vi "process_limits.vi"(10 "old output cluster":T1, 11 "Input cluster":T2) -> (0 "Update FPGA":bool, 3 "output cluster":T1)   [LabVIEW 2013]
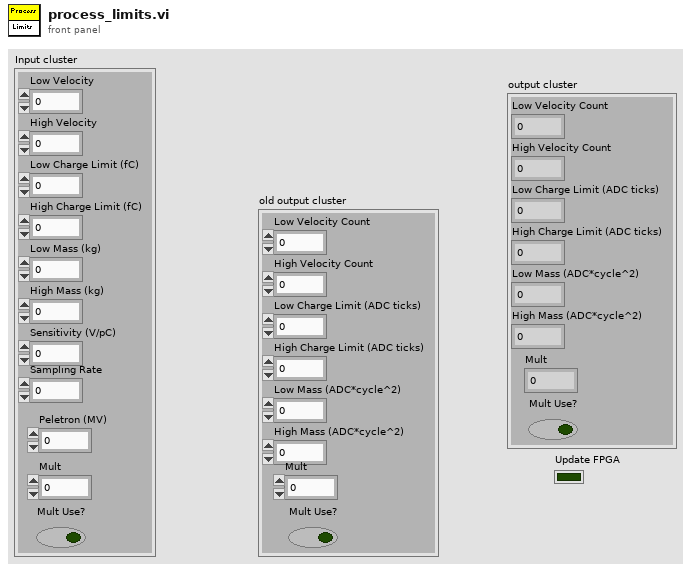
[diagram p1: front panel]
types:
  T1 = cluster{"Low Velocity Count":i32, "High Velocity Count":i32, "Low Charge Limit (ADC ticks)":i16, "High Charge Limit (ADC ticks)":i16, "Low Mass (ADC*cycle^2)":i64, "High Mass (ADC*cycle^2)":i64, "Mult":fxp<+,16,3>, "Mult Use?":bool}
  T2 = cluster{"Low Velocity":dbl, "High Velocity":dbl, "Low Charge Limit (fC)":dbl, "High Charge Limit (fC)":dbl, "Low Mass (kg)":dbl, "High Mass (kg)":dbl, "Sensitivity (V/pC)":dbl, "Sampling Rate":dbl, "Peletron (MV)":dbl, "Mult":fxp<+,16,3>, "Mult Use?":bool}
  T3 = cluster{"Low Velocity Count":i32, "High Velocity Count":i32, "Low Charge Limit (ADC ticks)":i16, "High Charge Limit (ADC ticks)":i16, "Low Mass (ADC*cycle^2)":i64, "High Mass (ADC*cycle^2)":i64}
  T4 = cluster{i32, i32, i16, i16, i64, i64, "Mult":fxp<+,16,3>, "Mult Use?":bool}
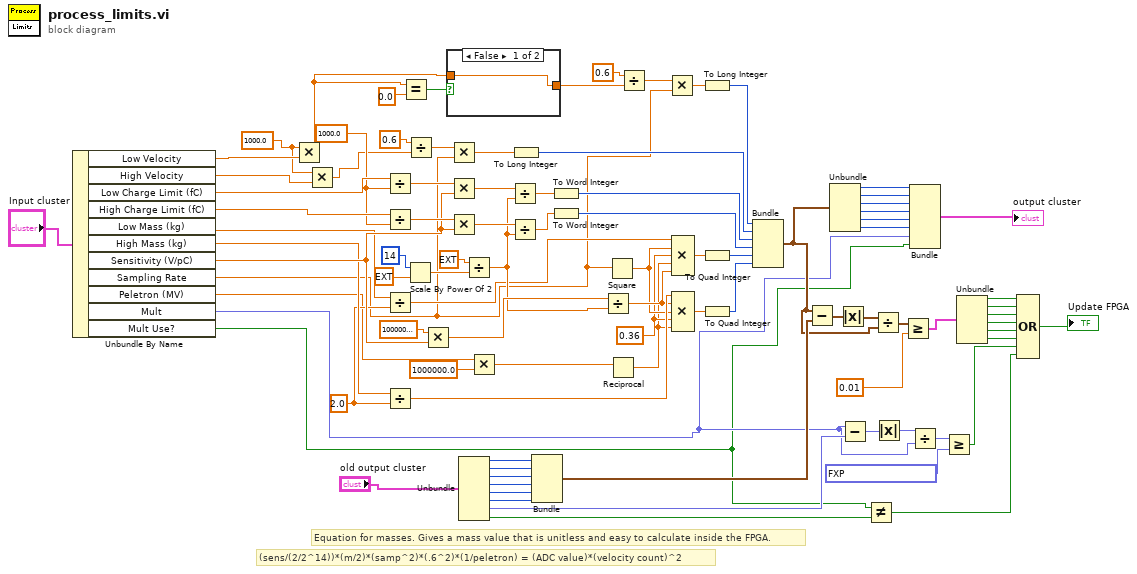
[diagram p0: block diagram]
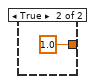
[diagram p2: hidden frame]
diagram:
  w41 = 1000.0 ("x")
  w50 = 0.36 ("value")
  w58 = 2.0 ("y")
  w71 = 1000.0 ("y")
  # "Equation for masses. Gives a mass value that is unitless and easy to calculate inside the FPGA."
  # "(sens/(2/2^14))*(m/2)*(samp^2)*(.6^2)*(1/peletron) = (ADC value)*(velocity count)^2"
  n1 = Unbundle By Name("Input cluster") -> ("Low Velocity"=w44:dbl, "High Velocity"=w42:dbl, "Low Charge Limit (fC)"=w79:dbl, "High Charge Limit (fC)"=w72:dbl, "Low Mass (kg)"=w60:dbl, "High Mass (kg)"=w59:dbl, "Sensitivity (V/pC)"=w64:dbl, "Sampling Rate"=w56:dbl, "Peletron (MV)"=w33:dbl, "Mult"=w8:fxp<+,16,3>, "Mult Use?"=w4:bool)
  n2 = Multiply(x=w41, y=w44) -> (x*y=w43:dbl)
  n3 = Multiply(x=w41, y=w42) -> (x*y=w40:dbl)
  n4 = Divide(x=w79, y=w71) -> (x/y=w78:dbl)
  n5 = Divide(x=w72, y=w71) -> (x/y=w70:dbl)
  n6 = Divide(x=w60, y=w58) -> (x/y=w57:dbl)
  n7 = Divide(x=w59, y=w58) -> (x/y=w53:dbl)
  n8 = Equal?(x=w43, y=0.0) -> (x = y?=w88:bool)
  n9 = Scale By Power Of 2(n=i16 14, x=ext 1.0) -> (x*2^n=w75:ext)
  n10 = Divide(x=0.6, y=w40) -> (x/y=w82:dbl)
  n11 = Multiply(x=1000000000000.0, y=w64) -> (x*y=w62:dbl)
  n12 = case shown="False" w88 {
    tunnel: [w92 1.0 ("y")] -> w87
    tunnel: w43 -> [w92 _]
    frame False {
    }
    frame True {
    }
  }
  n13 = Multiply(x=w82, y=w56) -> (x*y=w81:dbl)
  n14 = Multiply(x=w78, y=w64) -> (x*y=w69:dbl)
  n15 = Multiply(x=w70, y=w64) -> (x*y=w68:dbl)
  n16 = Unbundle("old output cluster") -> ("Low Velocity Count"=w26:i32, "High Velocity Count"=w25:i32, "Low Charge Limit (ADC ticks)"=w24:i16, "High Charge Limit (ADC ticks)"=w23:i16, "Low Mass (ADC*cycle^2)"=w22:i64, "High Mass (ADC*cycle^2)"=w21:i64, "Mult"=w11:fxp<+,16,3>, "Mult Use?"=w3:bool)
  n17 = Divide(x=ext 2.0, y=w75) -> (x/y=w61:ext)
  n18 = Multiply(x=w33, y=1000000.0) -> (x*y=w45:dbl)
  n19 = Divide(x=w69, y=w61) -> (x/y=w67:ext)
  n20 = Divide(x=w68, y=w61) -> (x/y=w66:ext)
  n21 = To Long Integer(number=w81) -> (32bit integer=w80:i32)
  n22 = Bundle("Low Velocity Count"=w26, "High Velocity Count"=w25, "Low Charge Limit (ADC ticks)"=w24, "High Charge Limit (ADC ticks)"=w23, "Low Mass (ADC*cycle^2)"=w22, "High Mass (ADC*cycle^2)"=w21) -> (w20:T3)  [unwired: 1 in]
  n23 = To Word Integer(number=w67) -> (16bit integer=w73:i16)
  n24 = To Word Integer(number=w66) -> (16bit integer=w65:i16)
  n25 = Divide(x=w62, y=w61) -> (x/y=w52:ext)
  n26 = Square(x=w56) -> (x^2=w51:dbl)
  n27 = Reciprocal(x=w45) -> (1/x=w49:dbl)
  n28 = Divide(x=0.6, y=w87) -> (x/y=w90:dbl)
  n29 = Multiply(x=w90, y=w56) -> (x*y=w85:dbl)
  n30 = Compound Arithmetic op=MULTIPLY(w57, w51, w50, w49, w52) -> (w55:ext)
  n31 = Compound Arithmetic op=MULTIPLY(w53, w52, w51, w50, w49) -> (w48:ext)
  n32 = To Long Integer(number=w85) -> (32bit integer=w84:i32)
  n33 = To Quad Integer(1:w55) -> (0:w54:i64)
  n34 = To Quad Integer(1:w48) -> (0:w47:i64)
  n35 = Bundle(w84, w80, w73, w65, w54, w47) -> (w19:cluster{i32, i32, i16, i16, i64, i64})  [unwired: 1 in]
  n36 = Subtract(x=w19, y=w20) -> (x-y=w32:cluster{i32, i32, i16, i16, i64, i64})
  n37 = Unbundle(w19) -> (w18:i32, w17:i32, w16:i16, w15:i16, w14:i64, w13:i64)
  n38 = Absolute Value(x=w32) -> (abs(x)=w31:cluster{i32, i32, i16, i16, i64, i64})
  n39 = Subtract(x=w8, y=w11) -> (x-y=w10:fxp<+/-,17,4>)
  n40 = Not Equal?(x=w4, y=w3) -> (x != y?=w2:bool)
  n41 = Divide(x=w31, y=w19) -> (x/y=w30:cluster{dbl, dbl, dbl, dbl, dbl, dbl})
  n42 = Absolute Value(x=w10) -> (abs(x)=w9:fxp<+,16,3>)
  n43 = Greater Or Equal?(x=w30, y=0.01) -> (x >= y?=w28:cluster{bool, bool, bool, bool, bool, bool})
  n44 = Bundle(w18, w17, w16, w15, w14, w13, "Mult"=w8, "Mult Use?"=w4) -> (→"output cluster":T4)  [unwired: 1 in]
  n45 = Divide(x=w9, y=w8) -> (x/y=w7:fxp<+,32,16>)
  n46 = Greater Or Equal?(x=w7, y=fxp<+,32,16> 0.0099945068359375) -> (x >= y?=w5:bool)
  n47 = Unbundle(w28) -> (w39:bool, w38:bool, w37:bool, w36:bool, w35:bool, w34:bool)
  n48 = Compound Arithmetic op=OR(w39, w38, w37, w36, w35, w34, w5, w2) -> (→"Update FPGA":bool)
